vi "XLP80_CAN_End.vi"(8 "err in":errorcluster caption="error") -> (0 "err out":errorcluster caption="error")   [LabVIEW 2021]
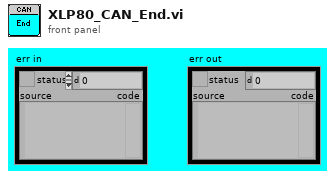
[diagram p1: front panel]
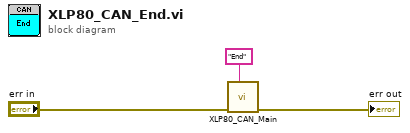
[diagram p0: block diagram]
diagram:
  n1 = call "XLP80_CAN_Main.vi"("Function"="End", "error in"="err in") -> ("error out"=→"err out":errorcluster)  [unwired: 9 in]
